vi "forceOutputState.vi"(8 "error in (no error)":errorcluster, 9 "calibratedValues":dbl[](array[numeric]), 10 "channel_addresses":string[](array[string]), 11 "HamegHMPSupply in":refnum<class "HamegHMPSupply.lvclass">) -> (0 "error out":errorcluster, 3 "HamegHMPSupply out":refnum<class "HamegHMPSupply.lvclass">)   [LabVIEW 2009, in "Hardware.lvlib" / "Channels.lvlib" / "HamegHMPSupply.lvclass"]
uses:
  HamegHMPSupply.lvclass
  HamegHMPSupply.lvclass/HamegHMPSupply.ctl
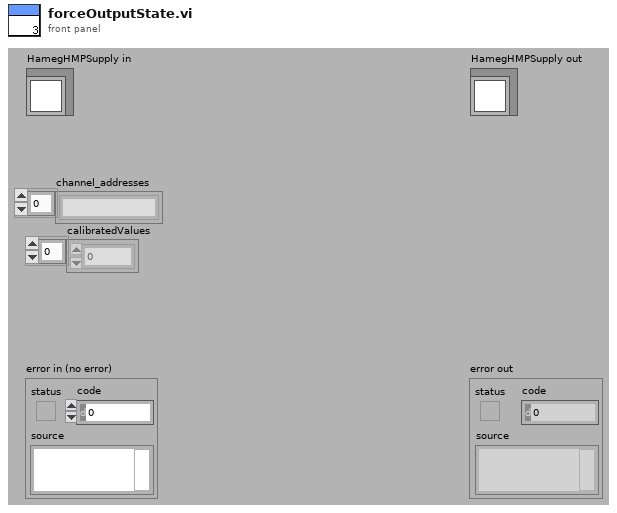
[diagram p1: front panel]
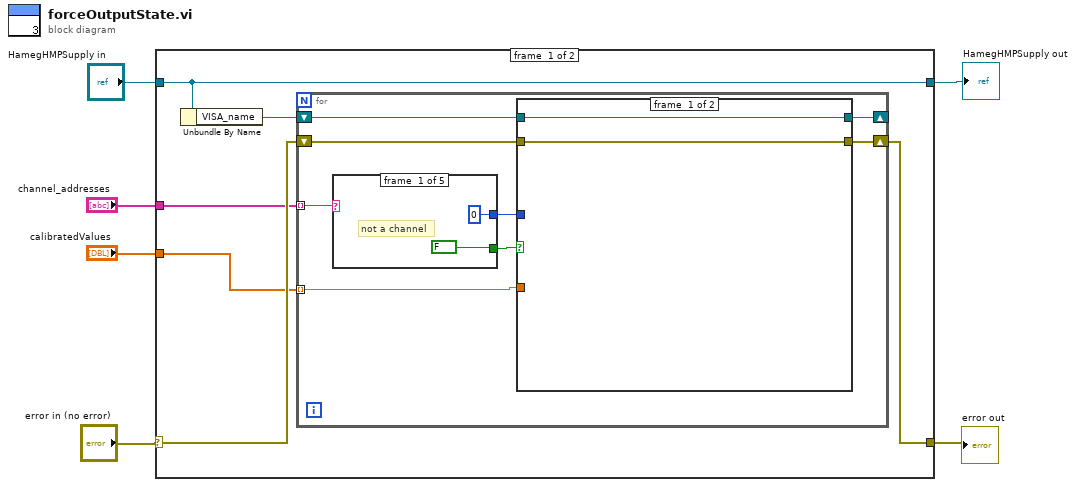
[diagram p0: block diagram]
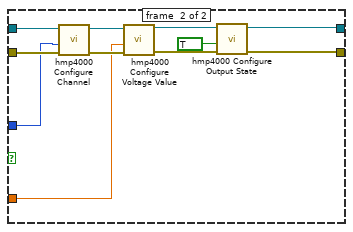
[diagram p2: hidden frame]
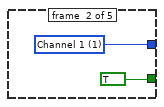
[diagram p3: hidden frame]
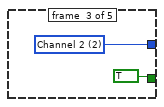
[diagram p4: hidden frame]
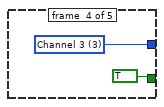
[diagram p5: hidden frame]
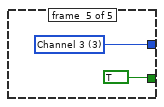
[diagram p6: hidden frame]
diagram:
  n1 = case shown="No Error" "error in (no error)" {
    selector: "error in (no error)" -> [w10 w44]
    tunnel: [w8 w44] -> w5
    tunnel: [w12 w45] -> w4
    tunnel: "HamegHMPSupply in" -> [w12 w45]
    tunnel: "channel_addresses" -> [w9 _]
    tunnel: "calibratedValues" -> [w7 _]
    frame #0 {
      n2 = Unbundle By Name(w12) -> ("VISA_name"=w11:refnum<visa-resource-name>)
      n3 = for {
        shift-right: [w15] -> _
        shift-left: w11 -> [w20]
        shift-right: [w14] -> w8
        shift-left: w10 -> [w19]
        tunnel: w9 -> [w18] mode=indexing
        tunnel: w7 -> [w13] mode=indexing
        n4 = case shown="\"Hameg2030_Ao_01\"" w18 {
          tunnel: [0 ("Channel (Channel 1)") w37 w39 w41 w43] -> w16
          tunnel: [FALSE TRUE TRUE TRUE TRUE] -> w17
          frame #0 {
            # "not a channel"
          }
          frame #1 {
            w37 = 1 items=["Channel 1"=1, "Channel 2"=2, "Channel 3"=3, "Channel 4"=4] ("Channel (Channel 1)")
          }
          frame #2 {
            w39 = 2 items=["Channel 1"=1, "Channel 2"=2, "Channel 3"=3, "Channel 4"=4] ("Channel (Channel 1)")
          }
          frame #3 {
            w41 = 3 items=["Channel 1"=1, "Channel 2"=2, "Channel 3"=3, "Channel 4"=4] ("Channel (Channel 1)")
          }
          frame #4 {
            w43 = 3 items=["Channel 1"=1, "Channel 2"=2, "Channel 3"=3, "Channel 4"=4] ("Channel (Channel 1)")
          }
        }
        n5 = case shown="True" w17 {
          tunnel: w20 -> [w22 w33]
          tunnel: w19 -> [w21 w32]
          tunnel: w16 -> [_ w31]
          tunnel: [w22 w24] -> w15
          tunnel: [w21 w23] -> w14
          tunnel: w13 -> [_ w27]
          frame #0 {
          }
          frame #1 {
            n6 = call <instrlib>:"hmp4000 Configure Channel.vi"("error in (no error)"=w32, "Channel (Channel 1)"=w31, "VISA resource name"=w33) -> ("error out"=w29:errorcluster, "VISA resource name out"=w30:refnum<visa-resource-name>)  [unwired: 7 in]
            n7 = call <instrlib>:"hmp4000 Configure Voltage Value.vi"("error in (no error)"=w29, "Voltage (0.0)"=w27, "VISA resource name"=w30) -> ("error out"=w25:errorcluster, "VISA resource name out"=w28:refnum<visa-resource-name>)  [unwired: 7 in]
            n8 = call <instrlib>:"hmp4000 Configure Output State.vi"("error in (no error)"=w25, "Output State (Off)"=TRUE, "VISA resource name"=w28) -> ("error out"=w23:errorcluster, "VISA resource name out"=w24:refnum<visa-resource-name>)  [unwired: 7 in]
          }
        }
      }
    }
    frame #1 {
    }
  }
  "error out" <- w5
  "HamegHMPSupply out" <- w4
